vi "GetPrivateQueueAction.vi"(8 "error in (no error)":errorcluster, 11 "DAQmx":refnum<class "DAQmx.lvclass">) -> (0 "error out":errorcluster, 2 "State":T1, 3 "DAQmx out":refnum<class "DAQmx.lvclass">)   [LabVIEW 2019, in "DAQmx.lvclass"]
uses:
  DAQmx.lvclass
  typedefs/DAQmx.States--enum.ctl
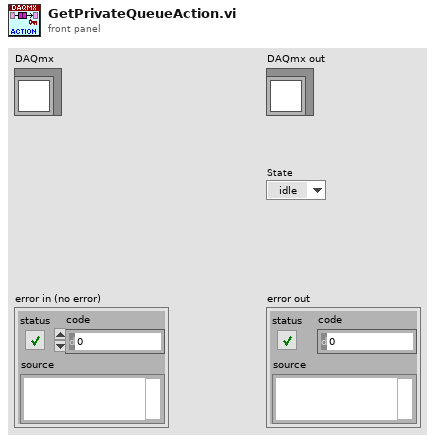
[diagram p1: front panel]
types:
  T1 = typedef "DAQmx.lvclass/DAQmx.States--enum.ctl" = enum16{"idle", "start", "stop", "calibrate", "auto", "exit"}
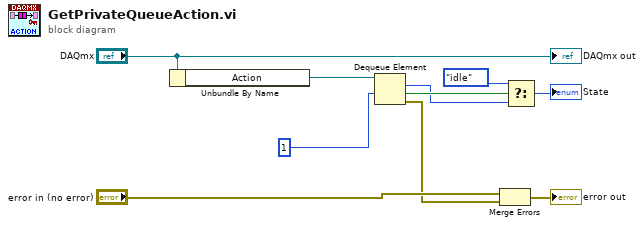
[diagram p0: block diagram]
diagram:
  n1 = Unbundle By Name("DAQmx") -> ("Action"=w8:refnum<queue>)
  n2 = Dequeue Element(queue=w8, timeout in ms (-1)=1) -> (element=w3:T1, timed out?=w7:bool, error out=w5:errorcluster)  [unwired: 1 in, 1 out]
  n3 = Merge Errors("error in (no error)", w5) -> (→"error out":errorcluster)
  n4 = Select(t=DAQmx.States--enum."idle", s=w7, f=w3) -> (s? t:f=→"State":T1)
  "DAQmx out" <- "DAQmx"
